vi "Teleop.vi"(10 "Match Info":T1={"Autonomous Elapsed Seconds"=0.0, "TeleOp Elapsed Seconds"=0.0, "Disabled Elapsed Seconds"=0.0, "Visited Autonomous"=FALSE, "Visited TeleOp"=FALSE, "Visited Disabled"=FALSE, "Autonomous Settings"={"Autonomous Style"=enum."Independent", "VI Refnum"=refnum}}, 11 "Call Context":T2) -> ()   [LabVIEW 2015]
doc: "This VI is called for each enabled TeleOp packet received from the DS. It is typically used to read from joysticks and other inputs and update I/O or setpoints for timed control loops. It should complete and return within 20 milliseconds or risk missing DS packets."
uses:
  <vilib>/Rock Robotics/WPI/DriverStation/WPI_DriverStationDerivedRobotMode.ctl
  <vilib>/Rock Robotics/WPI/DriverStation/WPI_DriverStationMatch Info.ctl
  <vilib>/Rock Robotics/WPI/Solenoid/WPI_SolenoidValue.ctl
  <vilib>/Rock Robotics/WPI/Utilities/WPI_GetSetVariantRefNum.vi
  <vilib>/Rock Robotics/Network Tables/NT Write Boolean Array.vi
  <vilib>/Rock Robotics/Network Tables/NT Write Numeric Array.vi
  <vilib>/Rock Robotics/WPI/Solenoid/Deprecated/WPI_SolenoidGetBool.vi
  <vilib>/Rock Robotics/WPI/RobotDrive/WPI_RobotDriveArcadeDrive_Standard(NoSaturation).vi
  <vilib>/Rock Robotics/WPI/Solenoid/WPI_SolenoidSetEnum.vi
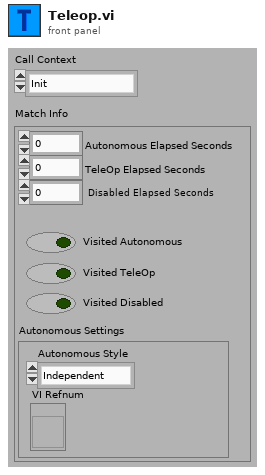
[diagram p1: front panel]
types:
  T1 = typedef "WPI_DriverStationMatch Info.ctl" = cluster{"Autonomous Elapsed Seconds":dbl, "TeleOp Elapsed Seconds":dbl, "Disabled Elapsed Seconds":dbl, "Visited Autonomous":bool, "Visited TeleOp":bool, "Visited Disabled":bool, "Autonomous Settings":cluster{"Autonomous Style":enum16{"Iterative", "Independent"}, "VI Refnum":refnum<vi>}}
  T2 = typedef "WPI_DriverStationDerivedRobotMode.ctl" = enum16{"Init", "Execute", "Stop"}
  T3 = typedef "WPI_SolenoidValue.ctl" = enum16{"Off", "On", "Forward", "Reverse"}
  T4 = typedef "WPI_JoystickDevRef.ctl" = cluster{"Device":T5}
  T5 = typedef "WPI_JoystickDeviceEnum.ctl" = enum16{"USB 0", "USB 1", "USB 2", "USB 3", "USB 4", "USB 5"}
  T6 = cluster{"Axes[0]":dbl, "Axes[1]":dbl, "Axes[2]":dbl, "Axes[3]":dbl, "Axes[4]":dbl, "Axes[5]":dbl, "Axes[6]":dbl, "Axes[7]":dbl, "Axes[8]":dbl}
  T7 = typedef "WPI_RobotDriveDevRef.ctl" = cluster{"DevStatus":errorcluster, "Motors[]":T8[], "Square Inputs":bool, "Max Output":dbl}
  T8 = typedef "WPI_MotorControlDeviceRef.ctl" = cluster{"DeviceStatus":errorcluster, "Type":T9, "PWM":cluster{"PWM Channel":T10, "DeadBand":T11}, "CAN":cluster{"Device Number":u8, "Control Mode":T12, "Semaphore":T13, "Max Vout":dbl, "TalonSRX Control Mode":T14}, "Invert":bool}
  T9 = typedef "WPI_MotorControlType.ctl" = enum16{"PWM", "CAN", "CANTalonSRX"}
  T10 = typedef "FPGA_DIOPWMChannel.ctl" = enum8{"PWM 0", "PWM 1", "PWM 2", "PWM 3", "PWM 4", "PWM 5", "PWM 6", "PWM 7", "PWM 8", "PWM 9", "PWM MXP 0", "PWM MXP 1", "PWM MXP 2", "PWM MXP 3", "PWM MXP 4", "PWM MXP 5", "PWM MXP 6", "PWM MXP 7", "PWM MXP 8", "PWM MXP 9", "Invalid"}
  T11 = typedef "WPI_PWMDeadband.ctl" = cluster{"Name":string, "maxPositivePwm":i32, "minPositivePwm":i32, "centerPwm":i32, "maxNegativePwm":i32, "minNegativePwm":i32, "angularRange":u16}
  T12 = typedef "WPI_CANJaguar_ControlMode.ctl" = enum8{"Percent VBus", "Current", "Speed", "Position", "Voltage"}
  T13 = typedef "Semaphore RefNum" = refnum<k1>
  T14 = typedef "WPI_CANTalonSRX_APIControlMode.ctl" = enum8{"Percent VBus", "Speed", "Position", "Slave", "Unchanged / Invalid", "Voltage Compensation", "Current", "Motion Profile"}
  T15 = typedef "WPI_SolenoidDevRef.ctl" = cluster{"DevStatus":errorcluster, "Pneumatics Control Module":u8, "Forward Solenoid Channel":T16, "Reverse Solenoid Channel":T16}
  T16 = typedef "WPI_SolenoidChannel.ctl" = enum8{"Solenoid 0", "Solenoid 1", "Solenoid 2", "Solenoid 3", "Solenoid 4", "Solenoid 5", "Solenoid 6", "Solenoid 7", "Invalid"}
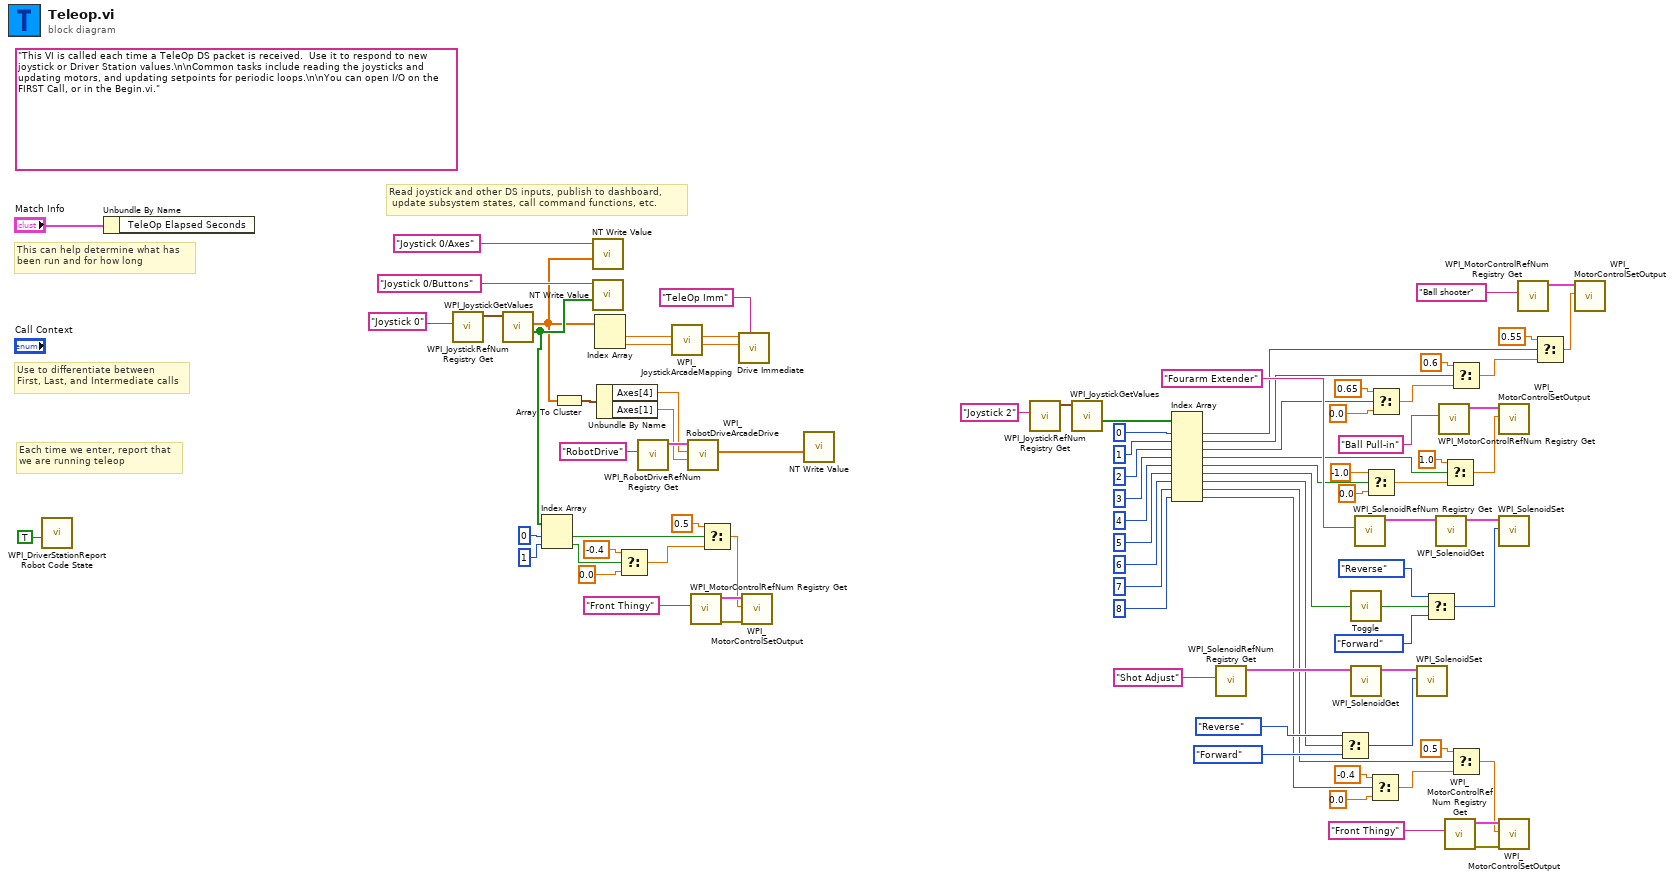
[diagram p0: block diagram]
diagram:
  (unwired) "This VI is called each time a TeleOp DS packet is received.  Use it to respond to new joystick or Driver Station values.\n\nCommon tasks include reading the joysticks and updating motors, and updating setpoints for periodic loops.\n\nYou can open I/O on the FIRST Call, or in the Begin.vi."
  # "Read joystick and other DS inputs, publish to dashboard,\n update subsystem states, call command functions, etc."
  # "Each time we enter, report that\nwe are running teleop"
  # "Use to differentiate between\nFirst, Last, and Intermediate calls"
  # "This can help determine what has\nbeen run and for how long"
  n1 = call <vilib>:"WPI_DriverStationReport Robot Code State.vi"("TeleOp"=TRUE ("Autonomous")) -> ()  [unwired: 10 in, 1 out]
  n2 = Unbundle By Name("Match Info") -> ()  [unwired: 1 out]
  n3 = call <vilib>:"WPI_JoystickRefNum Registry Get.vi"("refnum name"="Joystick 0") -> ("JoystickDevRef"=w86:T4)  [unwired: 1 in, 9 out]
  n4 = call <vilib>:"WPI_JoystickGetValues.vi"("JoystickDevRef"=w86) -> ("Buttons"=w65:bool[], "Axes"=w51:dbl[])  [unwired: 6 in, 3 out]
  n5 = Index Array(array=w65, index #1=0 ("index"), index #2=1 ("index")) -> (element #1=w3:bool, element #2=w2:bool)
  n6 = Array To Cluster(array=w51) -> (cluster=w52:T6)
  n7 = call-poly <vilib>:"NT Write Value.vi"("Numeric Array"=w51, "Name"="Joystick 0/Axes") -> ()  [unwired: 9 in, 1 out]
  n8 = call-poly <vilib>:"NT Write Value.vi"("Boolean Array"=w65, "Name"="Joystick 0/Buttons") -> ()  [unwired: 9 in, 1 out]
  n9 = Index Array(array=w51) -> (element #1=w82:dbl, element #2=w81:dbl)  [unwired: 2 in]
  n10 = Unbundle By Name(w52) -> ("Axes[4]"=w50:dbl, "Axes[1]"=w49:dbl)
  n11 = Select(t=-0.4, s=w2, f=0.0) -> (s? t:f=w62:dbl)
  n12 = call <vilib>:"WPI_RobotDriveRefNum Registry Get.vi"("refnum name"="RobotDrive" ("Name")) -> ("RobotDriveDevRef"=w55:T7)  [unwired: 9 in, 1 out]
  n13 = call <vilib>:"WPI_JoystickArcadeMapping.vi"("Y axis value"=w81, "X axis value"=w82) -> ("Right Motor Value"=w83:dbl, "Left Motor Value"=w84:dbl)  [unwired: 8 in]
  n14 = call-poly <vilib>:"WPI_RobotDriveArcadeDrive.vi"("Y axis value"=w49, "X axis value"=w50, "RobotDriveDevRef"=w55) -> ("Motor Values"=w53:dbl[])  [unwired: 6 in, 2 out]
  n15 = call <vilib>:"WPI_MotorControlRefNum Registry Get.vi"("refnum name"="Front Thingy") -> ("error out"=w57:errorcluster, "MotorControlDevRef"=w58:T8)  [unwired: 9 in]
  n16 = Select(t=0.5, s=w3, f=w62) -> (s? t:f=w56:dbl)
  n17 = call "Drive Immediate.vi"("Description"="TeleOp Imm", "Right Setpoint"=w83, "Left Setpoint"=w84) -> ()  [unwired: 8 in, 1 out]
  n18 = call <vilib>:"WPI_MotorControlSetOutput.vi"("error in (no error)"=w57, "Output"=w56, "MotorControlDevRef"=w58) -> ()  [unwired: 6 in, 3 out]
  n19 = call-poly <vilib>:"NT Write Value.vi"("Numeric Array"=w53) -> ()  [unwired: 10 in, 1 out]
  n20 = call <vilib>:"WPI_JoystickRefNum Registry Get.vi"("refnum name"="Joystick 2") -> ("JoystickDevRef"=w71:T4)  [unwired: 9 in, 1 out]
  n21 = call <vilib>:"WPI_JoystickGetValues.vi"("JoystickDevRef"=w71) -> ("Buttons"=w78:bool[])  [unwired: 6 in, 4 out]
  n22 = Index Array(array=w78, index #1=0 ("index"), index #2=1 ("index"), index #3=2 ("index"), index #4=3 ("index"), index #5=4 ("index"), index #6=5 ("index"), index #7=6 ("index"), index #8=7 ("index"), index #9=8 ("index")) -> (element #1=w45:bool, element #2=w37:bool, element #3=w36:bool, element #4=w33:bool, element #5=w32:bool, element #6=w25:bool, element #7=w14:bool, element #8=w10:bool, element #9=w8:bool)
  n23 = call <vilib>:"WPI_SolenoidRefNum Registry Get.vi"("refnum name"="Shot Adjust") -> ("SolenoidDevRef"=w19:T15)  [unwired: 9 in, 1 out]
  n24 = Select(t=WPI_SolenoidValue."Reverse" ("Value"), s=w14, f=WPI_SolenoidValue."Forward" ("Value")) -> (s? t:f=w13:T3)
  n25 = call "Toggle.vi"("Input"=w25) -> ("Toggled Output"=w24:bool)
  n26 = call-poly <vilib>:"WPI_SolenoidGet.vi"("SolenoidDevRef"=w19) -> ("SolenoidDevRef"=w20:T15)  [unwired: 8 in, 2 out]
  n27 = call <vilib>:"WPI_SolenoidRefNum Registry Get.vi"("refnum name"="Fourarm Extender") -> ("SolenoidDevRef"=w75:T15)  [unwired: 9 in, 1 out]
  n28 = Select(t=-1.0, s=w32, f=0.0) -> (s? t:f=w30:dbl)
  n29 = Select(t=-0.4, s=w8, f=0.0) -> (s? t:f=w9:dbl)
  n30 = Select(t=0.65, s=w36, f=0.0) -> (s? t:f=w41:dbl)
  n31 = call-poly <vilib>:"WPI_SolenoidSet.vi"("Value"=w13, "SolenoidDevRef"=w20) -> ()  [unwired: 8 in, 2 out]
  n32 = Select(t=WPI_SolenoidValue."Reverse" ("Value"), s=w24, f=WPI_SolenoidValue."Forward" ("Value")) -> (s? t:f=w67:T3)
  n33 = call-poly <vilib>:"WPI_SolenoidGet.vi"("SolenoidDevRef"=w75) -> ("SolenoidDevRef"=w73:T15)  [unwired: 8 in, 2 out]
  n34 = call <vilib>:"WPI_MotorControlRefNum Registry Get.vi"("refnum name"="Ball Pull-in") -> ("MotorControlDevRef"=w34:T8)  [unwired: 9 in, 1 out]
  n35 = Select(t=1.0, s=w33, f=w30) -> (s? t:f=w28:dbl)
  n36 = call <vilib>:"WPI_MotorControlRefNum Registry Get.vi"("refnum name"="Front Thingy") -> ("error out"=w23:errorcluster, "MotorControlDevRef"=w22:T8)  [unwired: 9 in]
  n37 = Select(t=0.6, s=w37, f=w41) -> (s? t:f=w43:dbl)
  n38 = Select(t=0.5, s=w10, f=w9) -> (s? t:f=w4:dbl)
  n39 = call <vilib>:"WPI_MotorControlSetOutput.vi"("Output"=w28, "MotorControlDevRef"=w34) -> ()  [unwired: 7 in, 3 out]
  n40 = call-poly <vilib>:"WPI_SolenoidSet.vi"("Value"=w67, "SolenoidDevRef"=w73) -> ()  [unwired: 8 in, 2 out]
  n41 = call <vilib>:"WPI_MotorControlSetOutput.vi"("error in (no error)"=w23, "Output"=w4, "MotorControlDevRef"=w22) -> ()  [unwired: 6 in, 3 out]
  n42 = call <vilib>:"WPI_MotorControlRefNum Registry Get.vi"("refnum name"="Ball shooter") -> ("MotorControlDevRef"=w47:T8)  [unwired: 9 in, 1 out]
  n43 = Select(t=0.55, s=w45, f=w43) -> (s? t:f=w38:dbl)
  n44 = call <vilib>:"WPI_MotorControlSetOutput.vi"("Output"=w38, "MotorControlDevRef"=w47) -> ()  [unwired: 7 in, 3 out]
